vi "SlewRateLimiter_SetRate.vi"(6 "NegativeRate":dbl=1.0, 9 "PositiveRate":dbl, 11 "in SLEW_RATE_LIMITER":T1 {"NegativeRateLimit" format="%13.5p"; "PrevTime" format="%30.5p"; "PrevValue" format="%13.5p"; "PositiveRateLimit" format="%13.5p"}) -> (3 "out SLEW_RATE_LIMITER":T1 {"NegativeRateLimit" format="%13.5p"; "PrevTime" format="%30.5p"; "PrevValue" format="%13.5p"; "PositiveRateLimit" format="%13.5p"})   [LabVIEW 2019, in "Trajectory_Library.lvlib"]
doc: "Sets the current rate value.\n\nInputs:\n - in Slew Rate Limiter -- The Slew Rate Limiter data cluster\n - Positive Rate -- The new positive rate limit in units/second. This is expected to be >= 0.\n - Negative Rate -- The new negative rate limit in units/second. This is expected to be <= 0. Optional. If not wired or the value is > 0 then the Positive Rate * -1 is used.\n \nOutputs:\n - out Slew Rate Limiter -- The modified Slew Rate Limiter data cluster"
uses:
  Trajectory_Library.lvlib
  TypeDef/SLEW_RATE_LIMITER.ctl
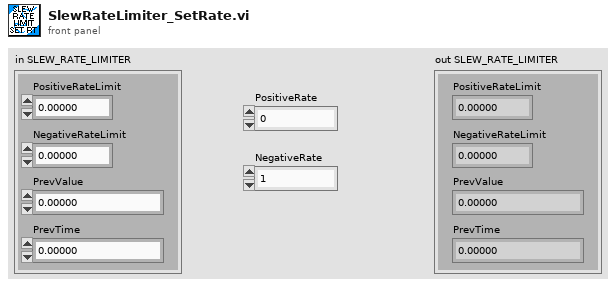
[diagram p1: front panel]
types:
  T1 = typedef "Trajectory_Library.lvlib/SLEW_RATE_LIMITER.ctl" = cluster{"PositiveRateLimit":dbl, "PrevValue":dbl, "PrevTime":dbl, "NegativeRateLimit":dbl}
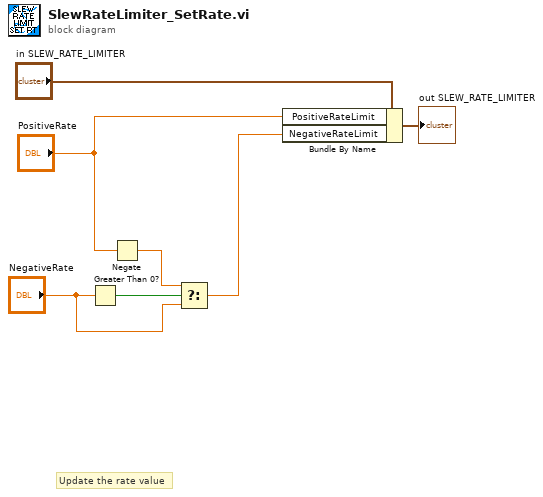
[diagram p0: block diagram]
diagram:
  # "Update the rate value"
  n1 = Greater Than 0?(x="NegativeRate") -> (x > 0?=w4:bool)
  n2 = Negate(x="PositiveRate") -> (-x=w3:dbl)
  n3 = Select(t=w3, s=w4, f="NegativeRate") -> (s? t:f=w1:dbl)
  n4 = Bundle By Name(cluster="in SLEW_RATE_LIMITER", "PositiveRateLimit"="PositiveRate", "NegativeRateLimit"=w1) -> (→"out SLEW_RATE_LIMITER":T1)
